vi "TimeConstantFilter_Example.vi"() -> ()   [LabVIEW 2019]
uses:
  <vilib>/Rock Robotics/WPI/ThirdParty/JAS_Junk/TrajLib/LinearFilter_ResetToValue.vi
  <vilib>/Rock Robotics/WPI/ThirdParty/JAS_Junk/TrajLib/LinearFilter_Calculate.vi
  <vilib>/Rock Robotics/WPI/ThirdParty/JAS_Junk/TrajLib/MathUtil_Clamp.vi
  <vilib>/Rock Robotics/WPI/ThirdParty/JAS_Junk/TrajLib/LinearFilter_MovingAverage.vi
  <vilib>/Rock Robotics/WPI/ThirdParty/JAS_Junk/TrajLib/LinearFilter_LowPassBW1.vi
  <vilib>/Rock Robotics/WPI/ThirdParty/JAS_Junk/TrajLib/LinearFilter_LowPassBW2.vi
  <vilib>/Rock Robotics/WPI/ThirdParty/JAS_Junk/TrajLib/LinearFilter_HighPassBW1.vi
  <vilib>/Rock Robotics/WPI/ThirdParty/JAS_Junk/TrajLib/LinearFilter_HighPassBW2.vi
  <vilib>/Rock Robotics/WPI/ThirdParty/JAS_Junk/TrajLib/Trajectory_Library.lvlib
panel:
  out "Wait Adjust":dbl format="%11.3f"
  in  "Auto / Manual":bool=TRUE
  in  "Enable\nNoise":bool=TRUE
  in  "Filter Enable":bool=TRUE
  in  "Use White Noise":bool=TRUE
  in  "Tab Control 2":T1(tab)
  out "LP BW 2":cluster{dbl, dbl, "Output_Value":dbl}(graph)
  out "Butter 1 Out":dbl format="%11.3f"
  out "Low Pass Butterworth 1 Dial":dbl(knob)=-2.895988890827539e-05 scale=-20.0..20.0
  out "Curoff Freq\nLP BW 1":dbl format="%11.3f"
  out "LP BW 2":cluster{dbl, dbl, "Output_Value":dbl}(graph)
  out "Butter 2 Out":dbl format="%11.3f"
  out "Low Pass Butterworth 2 Dial":dbl(knob)=-2.895988890827539e-05 scale=-20.0..20.0
  out "Cutoff  Freq\nLP BW 2":dbl format="%11.3f"
  out "Curoff Freq\nHP BW 1":dbl format="%11.3f"
  out "HP BW 1":cluster{dbl, dbl, "Output_Value":dbl}(graph)
  out "HP BW 1":dbl format="%11.3f"
  out "High Pass Butterworth 1":dbl(knob)=-2.895988890827539e-05 scale=-20.0..20.0
  out "HP  BW 2":cluster{dbl, dbl, "Output_Value":dbl}(graph)
  out "Alt Lag":dbl format="%11.3f"
  out "High Pass Butterworth 2":dbl(knob)=-2.895988890827539e-05 scale=-20.0..20.0
  out "Cutoff Freq\nHP BW 2":dbl format="%11.3f"
  out "Duration":dbl format="%11.3f"
  out "Late":dbl format="%11.3f"
  in  "Manual\nInput":dbl(slide) min=-12.0 max=12.0 scale=-12.0..12.0
  out "Raw Noise":dbl(knob)=-2.895988890827539e-05 scale=-20.0..20.0
  out "Raw Noise":dbl format="%11.3f"
  out "Actual Input":dbl(knob)=-2.895988890827539e-05 scale=-20.0..20.0
  out "Actual Input":dbl format="%11.3f"
  in  "Time Const (Sec)":dbl=0.08 min=0.0 step=0.001 format="%10.4f"
  out "Input":cluster{"Manual\nInput":dbl, dbl, "f":dbl}(graph)
  out "Meas Dial":dbl(knob)=-2.895988890827539e-05 scale=-20.0..20.0
  out "Measured Value":dbl format="%11.3f"
  # "Linear (Time Constant) Filter Example"
  # "Loop Information"
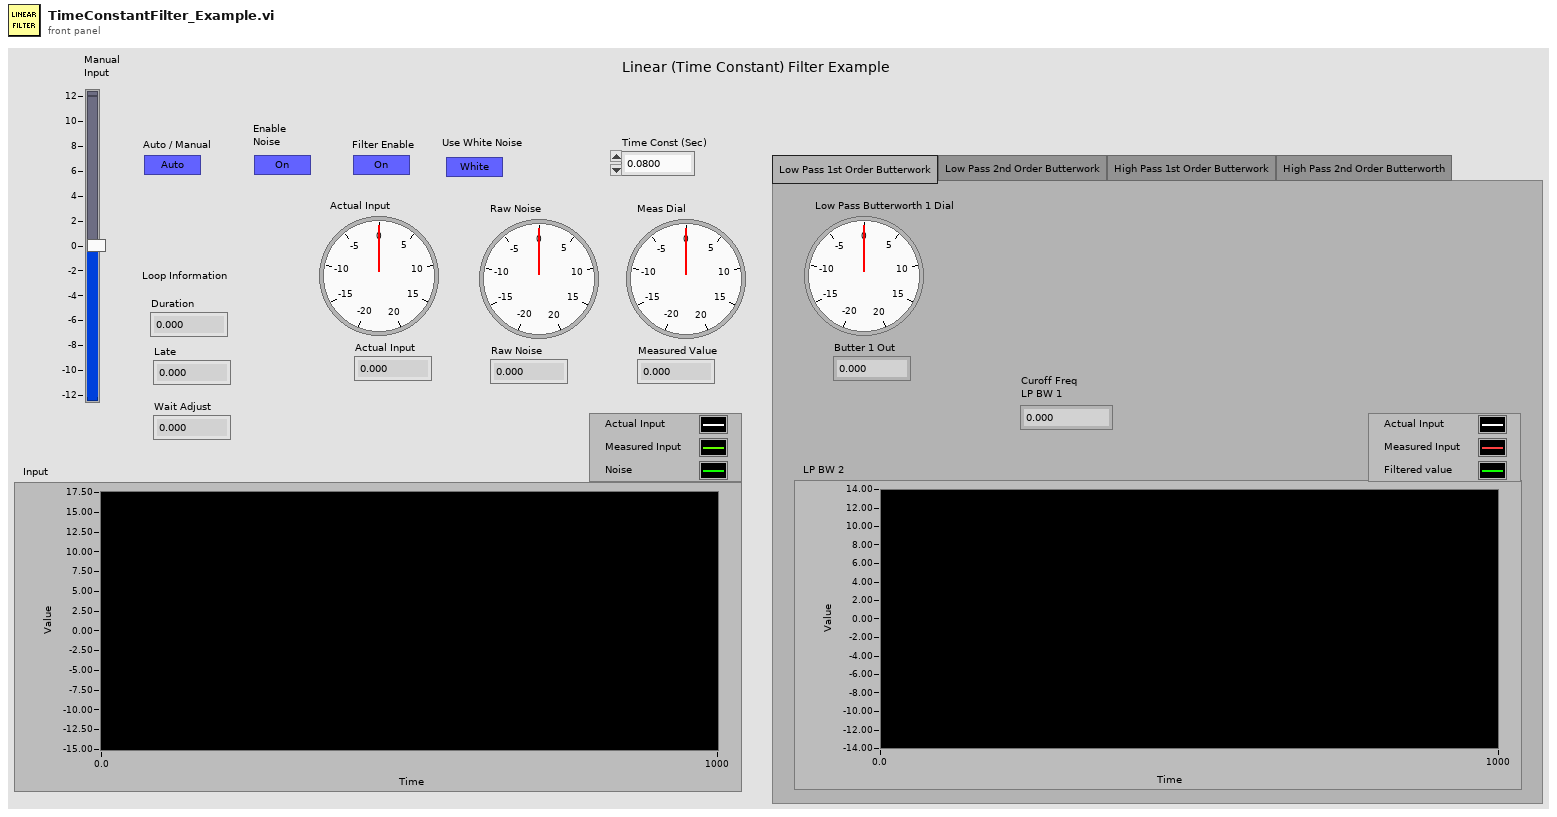
[diagram p1: front panel]
types:
  T1 = enum32{"Low Pass 1st Order Butterwork", "Low Pass 2nd Order Butterwork", "High Pass 1st Order Butterwork", "High Pass 2nd Order Butterworth"}
  T2 = enum16{"Moving Average", "Low Pass 1st Order Butterworth", "Low Pass 2nd Order Butterworth", "High Pass 1st Order Butterworth", "High Pass 2nd Order Butterworth"}
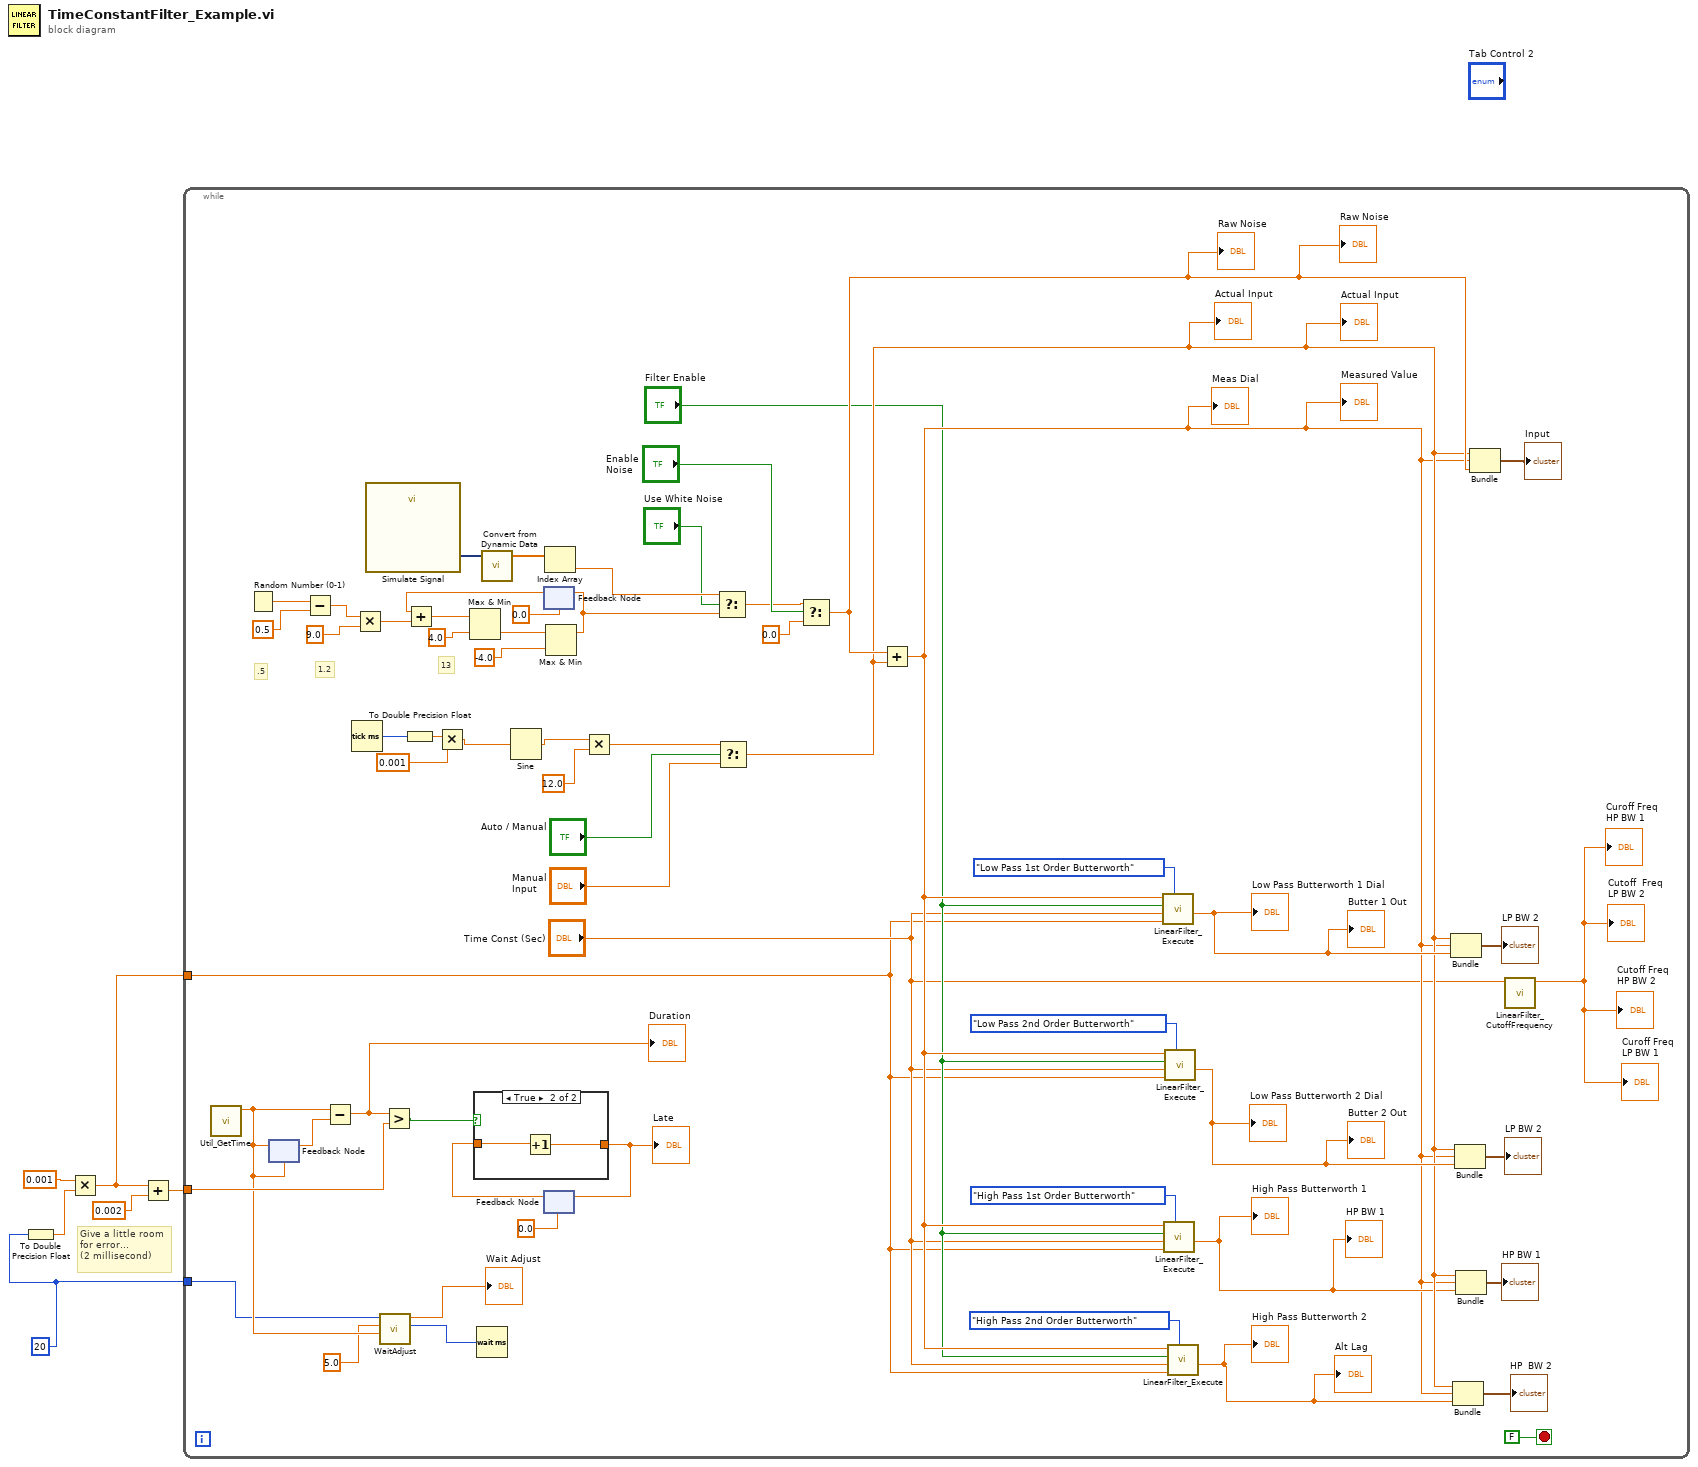
[diagram p0: block diagram]
diagram:
  w4 = u32 20 ("milliseconds to wait")
  # "Give a little room\nfor error...\n(2 millisecond)"
  n1 = To Double Precision Float(number=w4) -> (double precision float=w6:dbl)
  n2 = Multiply(x=0.001, y=w6) -> (x*y=w1:dbl)
  n3 = Add(x=w1, y=0.002) -> (x+y=w3:dbl)
  n4 = while {
    tunnel: w4 -> [w10]
    tunnel: w3 -> [w28]
    tunnel: w1 -> [w13]
    stop <- FALSE stop-if-true
    # "13"
    # "1.2"
    # ".5"
    n5 = call <vilib>:"Util_GetTime.vi"() -> ("FPGA_Time_Seconds"=w11:dbl)  [unwired: 10 in, 1 out]
    n6 = Random Number (0-1)() -> (number: 0 to 1=w62:dbl)
    n7 = feedback-in #1(w11) -> ()
    n8 = feedback #1(w11) -> (w31:dbl)
    n9 = Subtract(x=w62, y=0.5) -> (x-y=w58:dbl)
    n10 = Subtract(x=w11, y=w31) -> (x-y=w29:dbl)
    "Duration" <- w29
    n11 = Tick Count (ms)() -> (millisecond timer value=w55:u32)
    n12 = Multiply(x=w58, y=9.0) -> (x*y=w57:dbl)
    n13 = call "Simulate Signal"() -> ("DC with Uniform Noise"=w43:dynamicdata)  [unwired: 14 in, 1 out]
    n14 = call <vilib>:"WaitAdjust.vi"("Time_SEC"=w11, "MaxDeviation_MS"=5.0, "DesiredLoopTime_MS"=w10) -> ("AdjustedWaitTime_MS"=w8:u32, "Offset_MS"=→"Wait Adjust":dbl)  [unwired: 7 in]
    n15 = Greater?(x=w29, y=w28) -> (0:w30:bool)
    n16 = To Double Precision Float(number=w55) -> (double precision float=w56:dbl)
    n17 = Multiply(x=w56, y=0.001) -> (x*y=w53:dbl)
    n18 = Wait (ms)(milliseconds to wait=w8) -> ()  [unwired: 1 out]
    n19 = call "Convert from Dynamic Data"("Dynamic Data Type"=w43) -> ("Array"=w42:dbl[])  [unwired: 3 in]
    n20 = Sine(x=w53) -> (sin(x)=w52:dbl)
    n21 = feedback #2(0.0) -> (w59:dbl)
    n22 = Add(x=w59, y=w57) -> (x+y=w61:dbl)
    n23 = Max & Min(x=w61, y=4.0) -> (min(x,y)=w60:dbl)  [unwired: 1 out]
    n24 = feedback #3(0.0) -> (w36:dbl)
    n25 = case shown="True" w30 {
      tunnel: [w68 w70] -> w37
      tunnel: w36 -> [w68 w69]
      frame False {
      }
      frame True {
        n26 = Increment(x=w69) -> (x+1=w70:dbl)
      }
    }
    "Late" <- w37
    n27 = feedback-in #3(w37) -> ()
    n28 = Index Array(array=w42) -> (element=w41:dbl)  [unwired: 1 in]
    n29 = Max & Min(x=w60, y=-4.0) -> (max(x,y)=w44:dbl)  [unwired: 1 out]
    n30 = feedback-in #2(w44) -> ()
    n31 = Multiply(x=w52, y=12.0) -> (x*y=w49:dbl)
    n32 = Select(t=w41, s="Use White Noise", f=w44) -> (s? t:f=w45:dbl)
    n33 = Select(t=w49, s="Auto / Manual", f="Manual\nInput") -> (s? t:f=w21:dbl)
    "Actual Input" <- w21
    "Actual Input" <- w21
    n34 = Select(t=w45, s="Enable\nNoise", f=0.0) -> (s? t:f=w39:dbl)
    "Raw Noise" <- w39
    "Raw Noise" <- w39
    n35 = Add(x=w39, y=w21) -> (x+y=w16:dbl)
    "Measured Value" <- w16
    "Meas Dial" <- w16
    n36 = call <vilib>:"LinearFilter_Execute.vi"("Filter Type"=T2."Low Pass 1st Order Butterworth", "SamplePeriod"=w13, "TimeConstant"="Time Const (Sec)", "Enable"="Filter Enable", "Input"=w16) -> ("Output"=w27:dbl)  [unwired: 5 in, 1 out]
    "Butter 1 Out" <- w27
    "Low Pass Butterworth 1 Dial" <- w27
    n37 = call <vilib>:"LinearFilter_Execute.vi"("Filter Type"=T2."High Pass 1st Order Butterworth", "SamplePeriod"=w13, "TimeConstant"="Time Const (Sec)", "Enable"="Filter Enable", "Input"=w16) -> ("Output"=w17:dbl)  [unwired: 5 in, 1 out]
    "High Pass Butterworth 1" <- w17
    "HP BW 1" <- w17
    n38 = call <vilib>:"LinearFilter_Execute.vi"("Filter Type"=T2."Low Pass 2nd Order Butterworth", "SamplePeriod"=w13, "TimeConstant"="Time Const (Sec)", "Enable"="Filter Enable", "Input"=w16) -> ("Output"=w24:dbl)  [unwired: 5 in, 1 out]
    "Butter 2 Out" <- w24
    "Low Pass Butterworth 2 Dial" <- w24
    n39 = call <vilib>:"LinearFilter_Execute.vi"("Filter Type"=T2."High Pass 2nd Order Butterworth", "SamplePeriod"=w13, "TimeConstant"="Time Const (Sec)", "Enable"="Filter Enable", "Input"=w16) -> ("Output"=w18:dbl)  [unwired: 5 in, 1 out]
    "Alt Lag" <- w18
    "High Pass Butterworth 2" <- w18
    n40 = Bundle("Manual\nInput"=w21, w16, "Output"=w27) -> (→"LP BW 2":cluster{"Manual\nInput":dbl, dbl, "Output":dbl})  [unwired: 1 in]
    n41 = Bundle("Manual\nInput"=w21, w16, "Output"=w18) -> (→"HP  BW 2":cluster{"Manual\nInput":dbl, dbl, "Output":dbl})  [unwired: 1 in]
    n42 = Bundle("Manual\nInput"=w21, w16, "Output"=w24) -> (→"LP BW 2":cluster{"Manual\nInput":dbl, dbl, "Output":dbl})  [unwired: 1 in]
    n43 = Bundle("Manual\nInput"=w21, w16, "Output"=w17) -> (→"HP BW 1":cluster{"Manual\nInput":dbl, dbl, "Output":dbl})  [unwired: 1 in]
    n44 = Bundle("Manual\nInput"=w21, w16, "f"=w39) -> (→"Input":cluster{"Manual\nInput":dbl, dbl, "f":dbl})  [unwired: 1 in]
    n45 = call <vilib>:"LinearFilter_CutoffFrequency.vi"("TimeConstant"="Time Const (Sec)") -> ("Cutoff Freq"=→"Cutoff Freq\nHP BW 2" →"Curoff Freq\nLP BW 1" →"Cutoff  Freq\nLP BW 2" →"Curoff Freq\nHP BW 1":dbl)  [unwired: 10 in]
  }
